vi "Untitled 3.vi"() -> ()   [LabVIEW 2016]
uses:
  Global 1.vi
panel:
  in  "Stop Button 2":bool
  in  "Boolean 2":bool
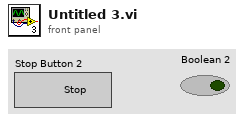
[diagram p1: front panel]
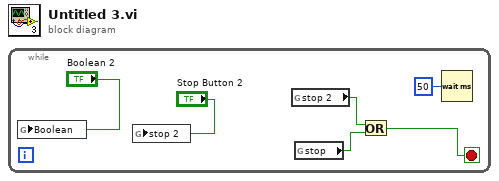
[diagram p0: block diagram]
diagram:
  n1 = while {
    stop <- w4 stop-if-true
    n2 = global write "Global 1.vi" "Boolean"("Boolean 2") -> ()
    n3 = global write "Global 1.vi" "stop 2"("Stop Button 2") -> ()
    n4 = global read "Global 1.vi" "stop 2"() -> (w3:bool)
    n5 = global read "Global 1.vi" "stop"() -> (w2:bool)
    n6 = Or(x=w3, y=w2) -> (x .or. y?=w4:bool)
    n7 = Wait (ms)(milliseconds to wait=u32 50) -> ()  [unwired: 1 out]
  }
